vi "Destroy.vi"(8 "error in (no error)":errorcluster, 11 "MeasurementServiceV2 in":refnum<class "MeasurementServiceV2.lvclass">) -> (0 "error out":errorcluster)   [LabVIEW 2020, in "MeasurementLink Measurement Server.lvlib" / "MeasurementServiceV2.lvclass"]
uses:
  MeasurementServiceV2.lvclass
  MeasurementServiceV2.lvclass/MeasurementServiceV2.ctl
  MeasurementLink Measurement Service Base V2/RPC Service/MeasurementService/MeasurementServiceBaseV2.lvclass
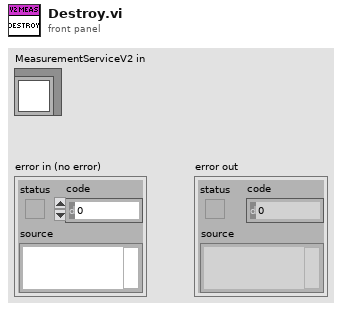
[diagram p1: front panel]
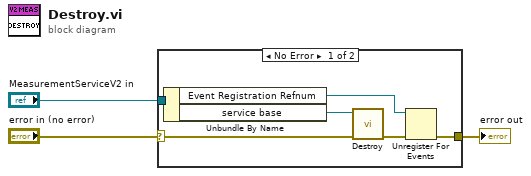
[diagram p0: block diagram]
diagram:
  n1 = case shown="No Error" "error in (no error)" {
    selector: "error in (no error)" -> [w7 w10]
    tunnel: [w5 w10] -> w2
    tunnel: "MeasurementServiceV2 in" -> [w9 _]
    frame No Error {
      n2 = Unbundle By Name(w9) -> ("Event Registration Refnum"=w4:refnum<event-registration>, "service base"=w8:refnum<class "MeasurementServiceBaseV2.lvclass">)
      n3 = call-dynamic "Destroy.vi"("error in (no error)"=w7, "SignalGeneratorService in"=w8) -> ("error out"=w6:errorcluster)  [unwired: 8 in, 1 out]
      n4 = Unregister For Events(event registration refnum=w4, error in=w6) -> (error out=w5:errorcluster)
    }
    frame Error {
    }
  }
  "error out" <- w2
